vi "[MDI] Child Set Parent.vi"(8 "error in (no error)":errorcluster, 9 "child":refnum<vi>, 10 "child name":string, 11 "[MDI] Parent in":refnum<class "[MDI] Parent.lvclass">) -> (0 "error out":errorcluster, 3 "[MDI] Parent out":refnum<class "[MDI] Parent.lvclass">)   [LabVIEW 2020, in "[MDI] Parent.lvlib" / "[MDI] Parent.lvclass"]
uses:
  [MDI] Parent.lvclass
  [MDI] Parent.lvclass/[MDI] Parent.ctl
  System.Windows.Forms
  user32.dll
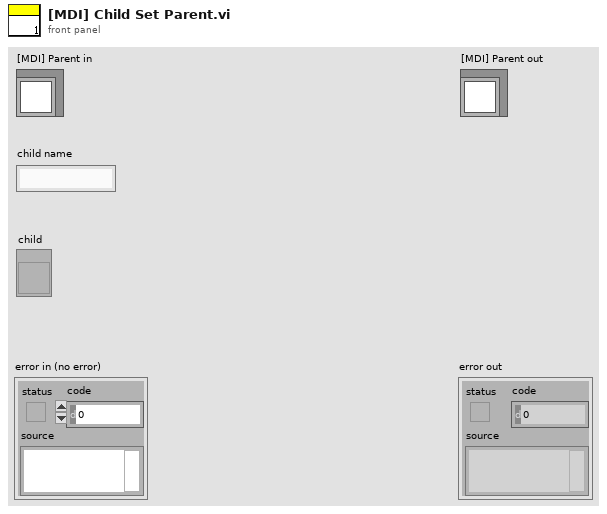
[diagram p1: front panel]
types:
  T1 = enum32{"Invalid", "Standard", "Closed", "Hidden", "Minimized", "Maximized"}
  T2 = typedef "LVRectTypeDef.ctl" = cluster{"Left":i16, "Top":i16, "Right":i16, "Bottom":i16}
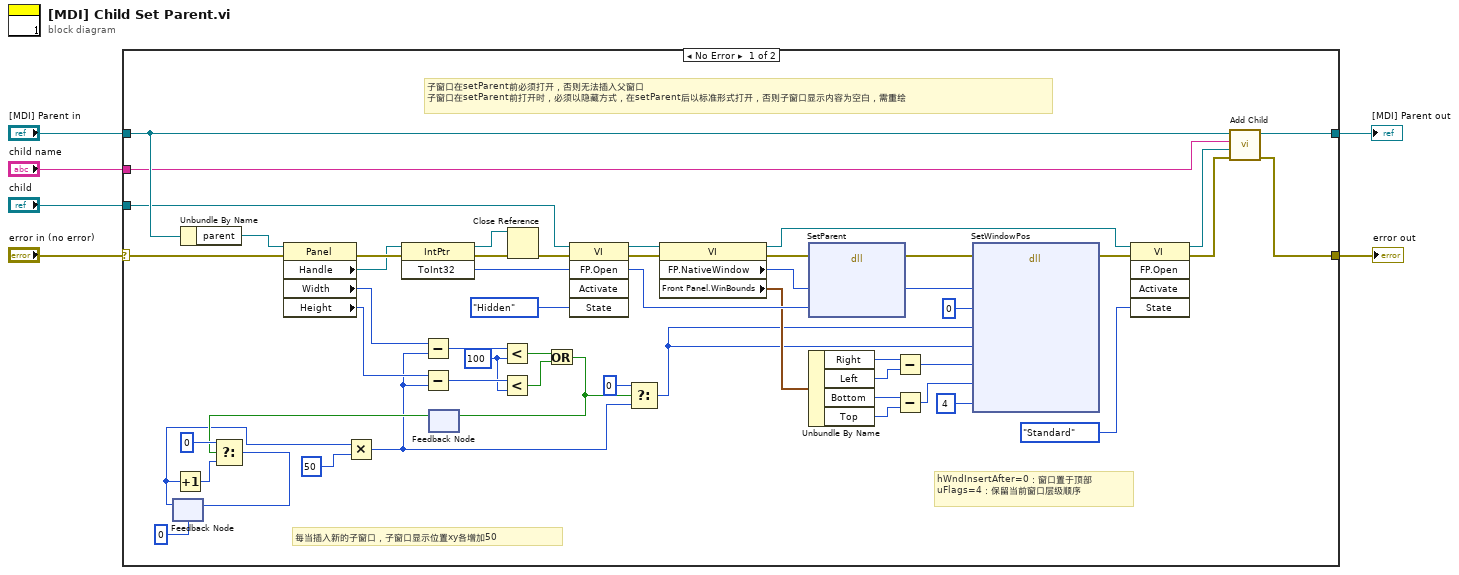
[diagram p0: block diagram]
diagram:
  n1 = case shown="No Error" "error in (no error)" {
    selector: "error in (no error)" -> [w52 w59]
    tunnel: [w10 w59] -> w4
    tunnel: [w13 w58] -> w3
    tunnel: "[MDI] Parent in" -> [w12 w58]
    tunnel: "child" -> [w11 _]
    tunnel: "child name" -> [w7 _]
    frame No Error {
      w37 = u32 100 ("y")
      # "子窗口在setParent前必须打开，否则无法插入父窗口\n子窗口在setParent前打开时，必须以隐藏方式，在setParent后以标准形式打开，否则子窗口显示内容为空白，需重绘"
      # "每当插入新的子窗口，子窗口显示位置xy各增加50"
      # "hWndInsertAfter=0：窗口置于顶部\nuFlags=4：保留当前窗口层级顺序"
      n2 = feedback #1(u32 0 ("hWndInsertAfter")) -> (w32:u32)
      n3 = Increment(x=w32) -> (x+1=w33:u32)
      n4 = Unbundle By Name(w12) -> ("parent"=w56:refnum<k24>)
      n5 = property class="Panel"(reference=w56, error in=w52) -> (error out=w57:errorcluster, "Handle"=w55:refnum<k24>, "Width"=w43:i32, "Height"=w42:i32)  [unwired: 1 out]
      n6 = Multiply(x=w32, y=u32 50) -> (x*y=w30:u32)
      n7 = invoke class="IntPtr" method="ToInt32"(reference=w55, error in=w57) -> (reference out=w50:refnum<k24>, error out=w51:errorcluster, "ToInt32"=w54:i32)  [unwired: 1 in]
      n8 = Subtract(x=w43, y=w30) -> (x-y=w39:u32)
      n9 = Subtract(x=w42, y=w30) -> (x-y=w38:u32)
      n10 = feedback #2() -> (w34:bool)  [unwired: 1 in]
      n11 = Select(t=u32 0, s=w34, f=w33) -> (s? t:f=w40:u32)
      n12 = feedback-in #1(w40) -> ()
      n13 = Less?(x=w39, y=w37) -> (x < y?=w36:bool)
      n14 = Less?(x=w38, y=w37) -> (x < y?=w35:bool)
      n15 = Close Reference(reference=w50, error in (no error)=w51) -> (error out=w48:errorcluster)
      n16 = Or(x=w36, y=w35) -> (x .or. y?=w31:bool)
      n17 = feedback-in #2(w31) -> ()
      n18 = invoke class="VI" method="FP.Open"(reference=w11, error in=w48, "State"=T1."Hidden") -> (error out=w47:errorcluster)  [unwired: 2 in, 4 out]
      n19 = Select(t=u32 0, s=w31, f=w30) -> (s? t:f=w29:u32)
      n20 = property class="VI"(reference=w11, error in=w47) -> (reference out=w26:refnum<vi>, error out=w49:errorcluster, "FP.NativeWindow"=w14:u64, "Front Panel.WinBounds"=w53:T2)
      n21 = dll-call lib="user32.dll" fn="SetParent"(error in=w49, "child"=w14, "newParent"=w54) -> (error out=w22:errorcluster, "child"=w24:u32)  [unwired: 4 in, 1 out]
      n22 = Unbundle By Name(w53) -> ("Right"=w20:i16, "Left"=w19:i16, "Bottom"=w18:i16, "Top"=w17:i16)
      n23 = Subtract(x=w20, y=w19) -> (x-y=w16:i16)
      n24 = Subtract(x=w18, y=w17) -> (x-y=w15:i16)
      n25 = dll-call lib="user32.dll" fn="SetWindowPos"(error in=w22, "hWnd"=w24, "hWndInsertAfter"=u32 0, "x"=w29, "y"=w29, "cx"=w16, "cy"=w15, "uFlags"=u32 4) -> (error out=w27:errorcluster)  [unwired: 10 in, 1 out]
      n26 = invoke class="VI" method="FP.Open"(reference=w26, error in=w27, "State"=T1."Standard") -> (reference out=w9:refnum<vi>, error out=w8:errorcluster)  [unwired: 2 in, 3 out]
      n27 = call "Add Child.vi"("error in (no error)"=w8, "child"=w9, "child name"=w7, "[MDI] Parent in"=w12) -> ("error out"=w10:errorcluster, "[MDI] Parent out"=w13:refnum<class "[MDI] Parent.lvclass">)  [unwired: 6 in]
    }
    frame Error {
    }
  }
  "error out" <- w4
  "[MDI] Parent out" <- w3
